vi "20150814 multi servo control.vi"(0 "Serial Port":refnum<visa-resource-name>="COM10", 1 "Action":T7(ring), 5 "LINX Resource in":T1, 7 "Servo Channels":u8[](array[numeric])=[2, 3, 4, 5, 6, 7, 8, 9, 10, 11, 12, 13], 9 "Pulse Widths (uS)":u16[](array[numeric])=[1500, 1500, 1500, 1500, 1500, 1500, 1500, 1500, 1500, 1500, 1500, 1500] min=600 max=2400 step=100, 11 "error in (no error)":errorcluster) -> (4 "Serial Port out":refnum<visa-resource-name>="COM10", 6 "LINX Resource out":T1, 8 "Servo initialize OK?":bool, 15 "Error Out":errorcluster)   [LabVIEW 2013]
uses:
  <vilib>/MakerHub/LINX/Private/Type Defs/LINX Ref.ctl
  <vilib>/MakerHub/LINX/Private/Type Defs/Platform.ctl
  <vilib>/MakerHub/LINX/Private/Type Defs/Interface.ctl
  <vilib>/MakerHub/LINX/Private/Device/Type Defs/LINX Device Config.ctl
  <vilib>/MakerHub/LINX/Private/Device/Type Defs/TCP Config.ctl
  <vilib>/MakerHub/LINX/Private/Device/Type Defs/Channels.ctl
  <vilib>/MakerHub/LINX/Public/Sensors/Motion/Servo/Servo Open N Channels.vi
  <vilib>/MakerHub/LINX/Public/Sensors/Motion/Servo/Servo Close N Channels.vi
  <vilib>/MakerHub/LINX/Public/Sensors/Motion/Servo/Servo Set Pulse Width N Channels.vi
  <vilib>/MakerHub/LINX/LMH-LINX.lvlib
  <vilib>/MakerHub/LINX/Public/Sensors/Motion/Servo/Servo.lvlib
  <vilib>/MakerHub/LINX/Private/Device/Device.lvlib
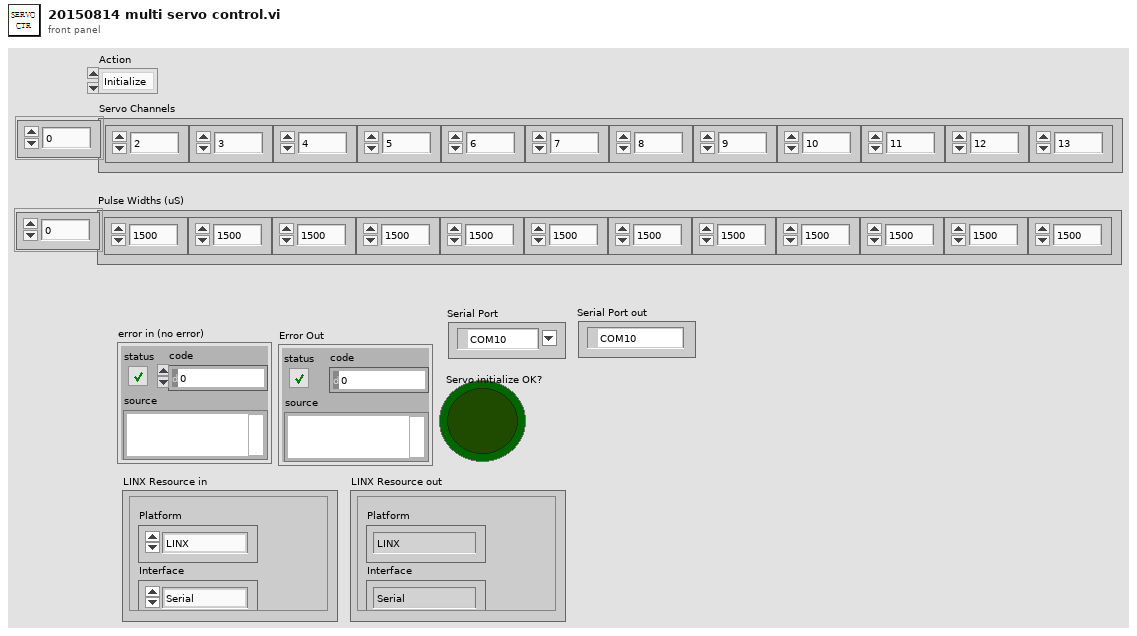
[diagram p1: front panel]
types:
  T1 = typedef "LMH-LINX.lvlib/LINX Ref.ctl" = cluster{"Platform":T2, "Interface":T3, "LINX Device Config":T4}
  T2 = typedef "LMH-LINX.lvlib/Platform.ctl" = enum16{"LINX", "myRIO"}
  T3 = typedef "LMH-LINX.lvlib/Interface.ctl" = enum16{"Serial", "TCP"}
  T4 = typedef "LMH-LINX.lvlib/Device.lvlib/LINX Device Config.ctl" = cluster{"Interface":T3, "COM Port":refnum<visa-resource-name>, "TCP Configuration":T5, "Device Family":u8, "Device ID":u8, "Device Name":string, "TCP Ref":refnum<k5>, "Channels":T6}
  T5 = typedef "LMH-LINX.lvlib/Device.lvlib/TCP Config.ctl" = cluster{"IP Address":string, "Port":u16}
  T6 = typedef "LMH-LINX.lvlib/Channels.ctl" = cluster{"DI":u8[], "DO":u8[], "AI":u8[], "AO":u8[], "PWM":u8[], "QE":u8[], "UART":u8[], "I2C 2":u8[], "SPI":u8[], "CAN":u8[], "Servo":u8[], "AI Ref (V)":dbl, "AO Ref (V)":dbl, "AO Resolution (Bits)":u8}
  T7 = enum16{"Initialize", "Close", "Set Pulse widths"}
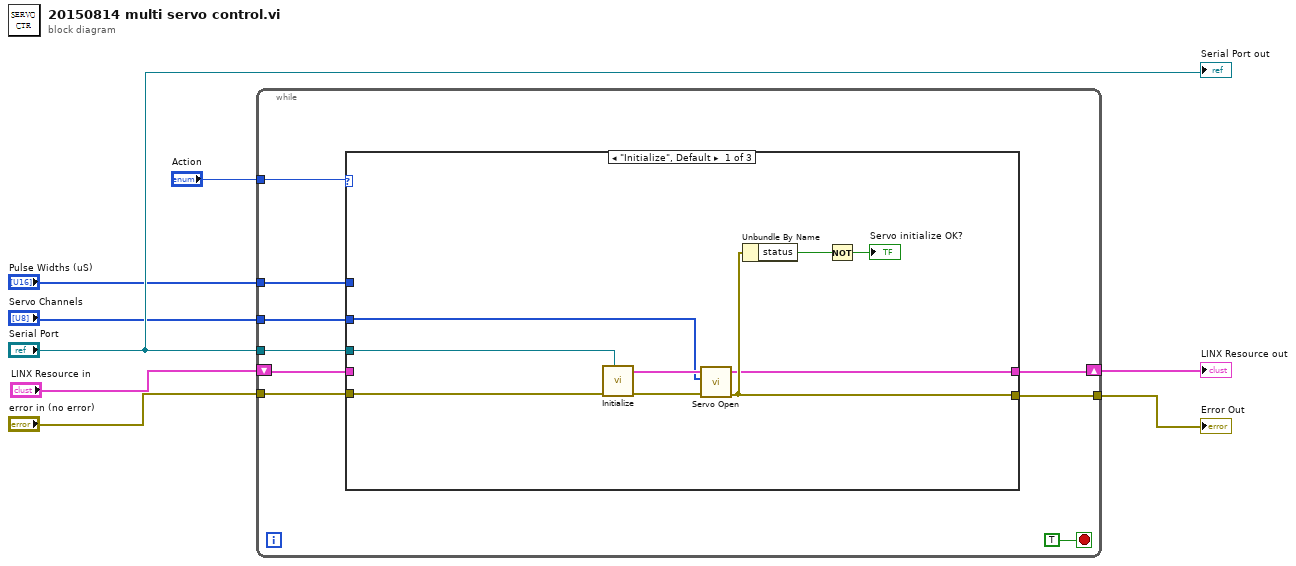
[diagram p0: block diagram]
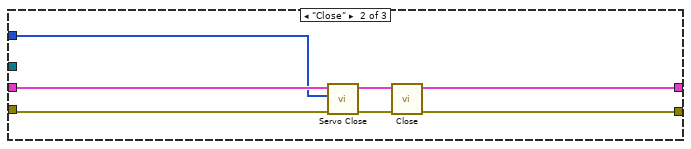
[diagram p2: hidden frame]
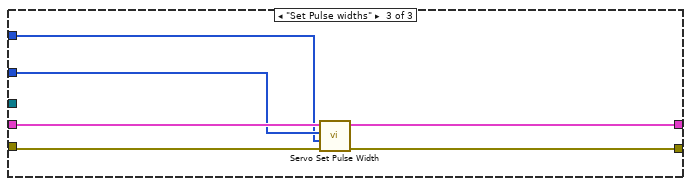
[diagram p3: hidden frame]
diagram:
  n1 = while {
    tunnel: "Action" -> [w17]
    tunnel: "error in (no error)" -> [w15]
    tunnel: [w14] -> w7
    tunnel: "Serial Port" -> [w13]
    tunnel: "Servo Channels" -> [w12]
    shift-right: [w11] -> w1
    shift-left: "LINX Resource in" -> [w10]
    tunnel: "Pulse Widths (uS)" -> [w9]
    stop <- TRUE stop-if-true
    n2 = case shown="\"Initialize\", Default" w17 {
      tunnel: w15 -> [w21 w30 w36]
      tunnel: [w22 w31 w35] -> w14
      tunnel: w13 -> [w20 _ _]
      tunnel: w12 -> [w19 w27 w37]
      tunnel: [w18 w28 w38] -> w11
      tunnel: w10 -> [_ w29 w39]
      tunnel: w9 -> [_ _ w34]
      frame "Initialize", Default {
        n3 = call <vilib>:"Initialize.vi"("Serial Port"=w20, "Error In"=w21) -> ("Error Out"=w26:errorcluster, "LINX Ref"=w25:T1)  [unwired: 7 in, 1 out]
        n4 = call-poly <vilib>:"Servo Open.vi"("Error In"=w26, "Servo Channels"=w19, "LINX Resource"=w25) -> ("Error Out"=w22:errorcluster, "LINX Resource"=w18:T1)  [unwired: 7 in]
        n5 = Unbundle By Name(w22) -> ("status"=w23:bool)
        n6 = Not(x=w23) -> (.not. x?=→"Servo initialize OK?":bool)
      }
      frame "Close" {
        n7 = call-poly <vilib>:"Servo Close.vi"("Error In"=w30, "Servo Channels"=w27, "LINX Resource"=w29) -> ("Error Out"=w32:errorcluster, "LINX Resource"=w33:T1)  [unwired: 7 in]
        n8 = call <vilib>:"Close.vi"("Error In"=w32, "LINX Resource"=w33) -> ("Error Out"=w31:errorcluster, "LINX Resource"=w28:T1)  [unwired: 8 in]
      }
      frame "Set Pulse widths" {
        n9 = call-poly <vilib>:"Servo Set Pulse Width.vi"("Error In"=w36, "Pulse Widths (uS)"=w34, "Servo Channels"=w37, "LINX Resource"=w39) -> ("Error Out"=w35:errorcluster, "LINX Resource"=w38:T1)  [unwired: 6 in]
      }
    }
  }
  "Error Out" <- w7
  "LINX Resource out" <- w1
  "Serial Port out" <- "Serial Port"
